vi "Tap Title Modflication.vi"(10 "Test Item Name":string[](array[string])=["SDD21", "SDD22", "SCD21", "SCD22", "SCC11", "SCC22", "NEXT", "FEXT"], 11 "Tab_Graph":refnum<vi>) -> ()   [LabVIEW 2011]
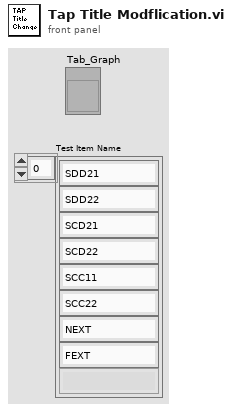
[diagram p1: front panel]
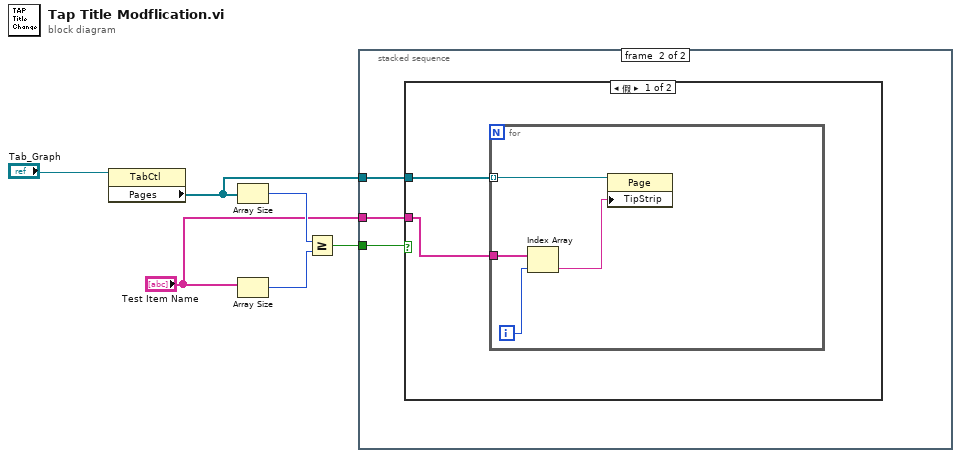
[diagram p0: block diagram]
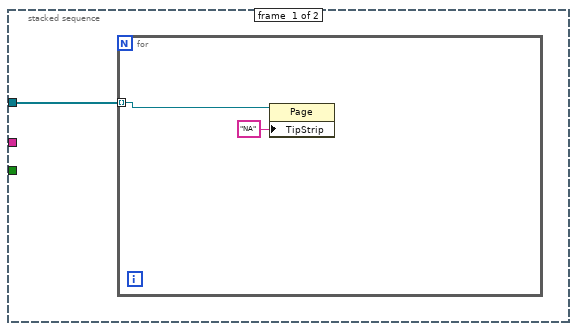
[diagram p2: hidden frame]
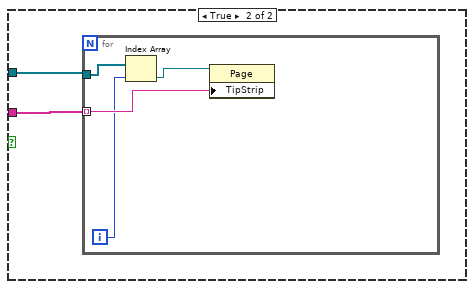
[diagram p3: hidden frame]
diagram:
  n1 = property class="TabCtl"(reference="Tab_Graph") -> ("Pages"=w2:refnum<vi>[])  [unwired: 1 in, 2 out]
  n2 = Array Size(array=w2) -> (size(s)=w6:i32)
  n3 = Array Size(array="Test Item Name") -> (size(s)=w5:i32)
  n4 = Greater Or Equal?(x=w6, y=w5) -> (x >= y?=w4:bool)
  n5 = stacked-sequence {
    tunnel: w4 -> [_ w12]
    tunnel: "Test Item Name" -> [_ w11]
    tunnel: w2 -> [w7 w10]
    frame #0 {
      n6 = for {
        tunnel: w7 -> [w9] mode=indexing
        n7 = property class="Page"(reference=w9, "TipStrip"="NA" ("提示框")) -> ()  [unwired: 1 in, 2 out]
      }
    }
    frame #1 {
      n8 = case shown="假" w12 {
        tunnel: w11 -> [w13 w20]
        tunnel: w10 -> [w14 w19]
        frame False {
          n9 = for {
            tunnel: w14 -> [w18] mode=indexing
            tunnel: w13 -> [w17]
            i -> [w16]
            n10 = Index Array(array=w17, index=w16) -> (element=w15:string)
            n11 = property class="Page"(reference=w18, "TipStrip"=w15) -> ()  [unwired: 1 in, 2 out]
          }
        }
        frame True {
          n12 = for {
            tunnel: w20 -> [w24] mode=indexing
            tunnel: w19 -> [w23]
            i -> [w22]
            n13 = Index Array(array=w23, index=w22) -> (element=w21:refnum<vi>)
            n14 = property class="Page"(reference=w21, "TipStrip"=w24) -> ()  [unwired: 1 in, 2 out]
          }
        }
      }
    }
  }
